vi "WritePayload(UDP).vi"(9 "Payload":u8[](array[numeric]), 11 "Ethernet Frame In":u8[](array[numeric]) format="%.0x") -> (3 "Ethernet Frame Out":u8[](array[numeric]) format="%.0x")   [LabVIEW 2020, in "EthFrameManagement.lvlib"]
doc: "Write the Payload in the Ethernet Frame."
uses:
  EthFrameManagement.lvlib
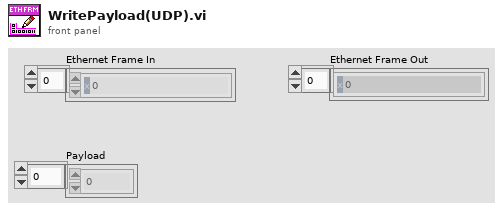
[diagram p1: front panel]
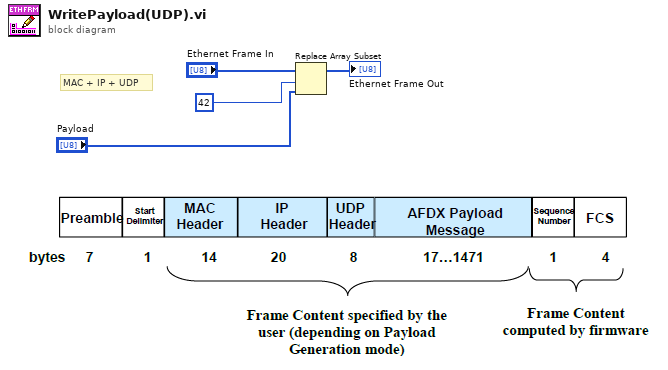
[diagram p0: block diagram]
diagram:
  # "MAC + IP + UDP"
  n1 = Replace Array Subset(array="Ethernet Frame In", new element="Payload", index=42) -> (→"Ethernet Frame Out":u8[])
